vi "Get State.vi"(8 "error in (no error)":errorcluster, 11 "Instrument Actor in":refnum<class "Instrument Actor.lvclass">) -> (0 "error out":errorcluster, 1 "Result ready":bool, 2 "Armed":bool, 3 "Instrument Actor out":refnum<class "Instrument Actor.lvclass">, 4 "Check again":bool)   [LabVIEW 2019, in "Instrument Actor.lvclass"]
uses:
  Instrument Actor.lvclass
  C:/GitHub/LabActor/Worker/Worker.lvclass
  Worker/Worker.lvclass/Worker.ctl
  Instrument Actor.lvclass/Instrument Actor.ctl
  Read Instrument driver.vi
  Worker/Read Cycle count.vi
  Worker/Write Cycle count.vi
  Write Instrument driver.vi
  Template Module/Read State.vi
  NHMFL_Core/Libraries/Instruments/Instrument Driver/Instrument Driver.lvclass
  Worker/Worker.lvclass
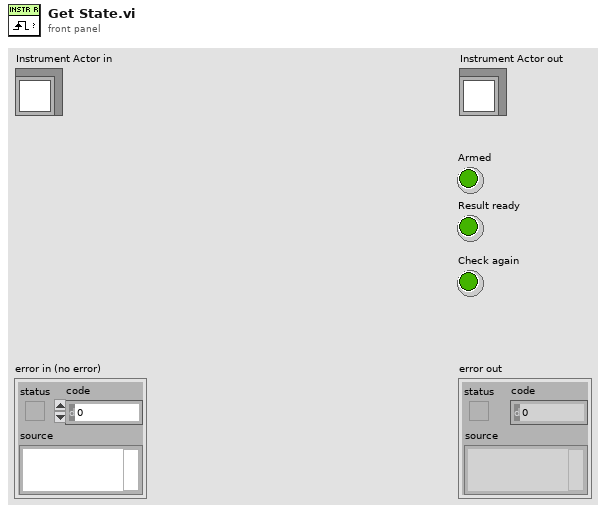
[diagram p1: front panel]
types:
  T1 = typedef "Worker State.ctl" = enum16{"Idle", "Starting", "Working", "Stopping"}
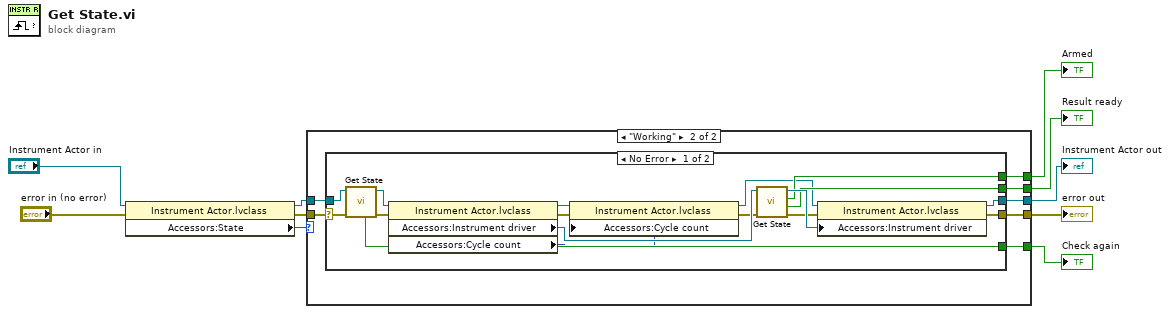
[diagram p0: block diagram]
diagram:
  n1 = property class="Instrument Actor.lvclass"(reference="Instrument Actor in", error in="error in (no error)") -> (reference out=w7:refnum<class "Instrument Actor.lvclass">, error out=w6:errorcluster, "Accessors:State"=w4:T1)
  n2 = case shown="\"Working\"" w4 {
    tunnel: [w11 w19] -> w10
    tunnel: [w12 w18] -> w9
    tunnel: w7 -> [w12 w17]
    tunnel: w6 -> [w11 w16]
    tunnel: [_ w15] -> w3
    tunnel: [_ w14] -> w2
    tunnel: [_ w13] -> w1
    frame "Idle", Default {
    }
    frame "Working" {
      n3 = case shown="No Error" w16 {
        selector: w16 -> [w35 w38]
        tunnel: [w31 w38] -> w19
        tunnel: [w30 w37] -> w18
        tunnel: w17 -> [w26 w37]
        tunnel: [w29 _] -> w15
        tunnel: [w28 _] -> w14
        tunnel: [w24 _] -> w13
        frame No Error {
          n4 = call-parent "Get State.vi"("error in (no error)"=w35, "Worker in"=w26) -> ("error out"=w27:errorcluster, "Worker out"=w25:refnum<class "Instrument Actor.lvclass">, "Check again"=w24:bool)  [unwired: 5 in, 2 out]
          n5 = property class="Instrument Actor.lvclass"(reference=w25, error in=w27) -> (reference out=w22:refnum<class "Instrument Actor.lvclass">, error out=w34:errorcluster, "Accessors:Instrument driver"=w36:refnum<class "Instrument Driver.lvclass">, "Accessors:Cycle count"=w20:i32)
          n6 = property class="Instrument Actor.lvclass"(reference=w22, error in=w34, "Accessors:Cycle count"=w20) -> (reference out=w21:refnum<class "Instrument Actor.lvclass">, error out=w23:errorcluster)
          n7 = call-dynamic "Get State.vi"("error in (no error)"=w23, "Instrument Driver in"=w36) -> ("error out"=w32:errorcluster, "Data ready"=w28:bool, "Armed"=w29:bool, "Instrument Driver out"=w33:refnum<class "Instrument Driver.lvclass">)  [unwired: 4 in, 2 out]
          n8 = property class="Instrument Actor.lvclass"(reference=w21, error in=w32, "Accessors:Instrument driver"=w33) -> (reference out=w30:refnum<class "Instrument Actor.lvclass">, error out=w31:errorcluster)
        }
        frame Error {
        }
      }
    }
  }
  "error out" <- w10
  "Instrument Actor out" <- w9
  "Armed" <- w3
  "Result ready" <- w2
  "Check again" <- w1
